vi "Read Model.vi"(8 "error in":errorcluster, 11 "Configurable Device in":refnum<class "Configurable Device.lvclass">) -> (0 "error out":errorcluster, 2 "Model":string, 3 "Configurable Device out":refnum<class "Configurable Device.lvclass">)   [LabVIEW 2016, in "Configurable Device.lvclass"]
uses:
  Configurable Device.lvclass
  Configurable Device.lvclass/Configurable Device.ctl
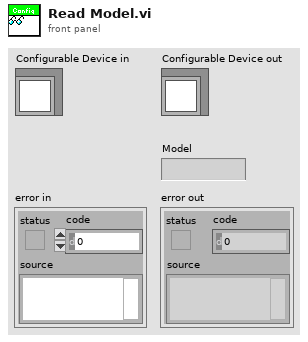
[diagram p1: front panel]
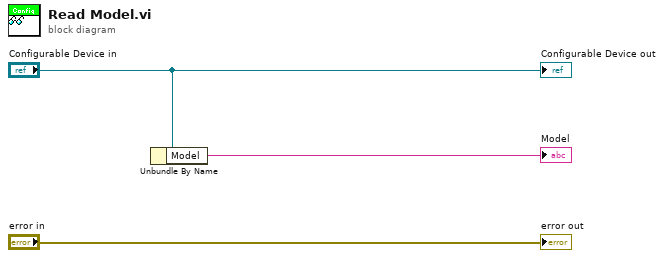
[diagram p0: block diagram]
diagram:
  n1 = Unbundle By Name("Configurable Device in") -> ("Model"=→"Model":string)
  "error out" <- "error in"
  "Configurable Device out" <- "Configurable Device in"
